vi "Utils.vi"(8 "error in":errorcluster, 10 "Data":variant, 11 "Command":string) -> (0 "error out":errorcluster, 3 "Return Data":variant)   [LabVIEW 2014]
uses:
  <vilib>/Utility/traverseref.llb/TRef TravTarget.ctl
  <vilib>/Utility/traverseref.llb/VI Scripting - Traverse.lvlib
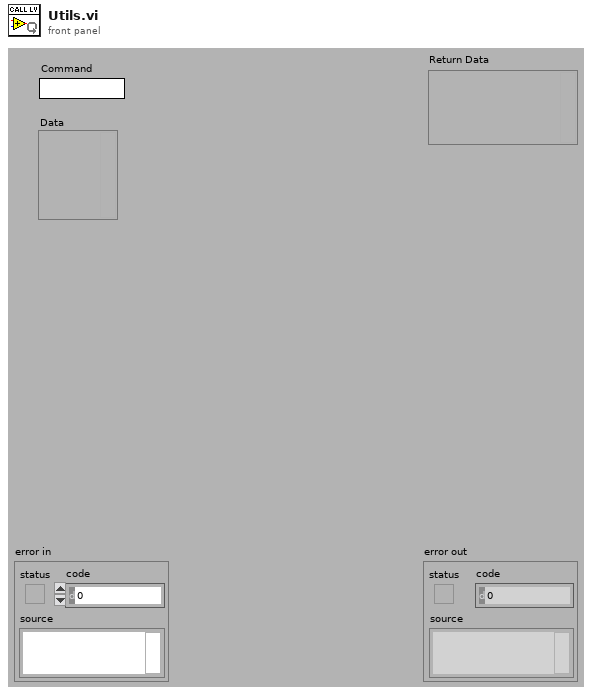
[diagram p1: front panel]
types:
  T1 = typedef "TRef TravTarget.ctl" = enum16{"FP", "BD", "Other"}
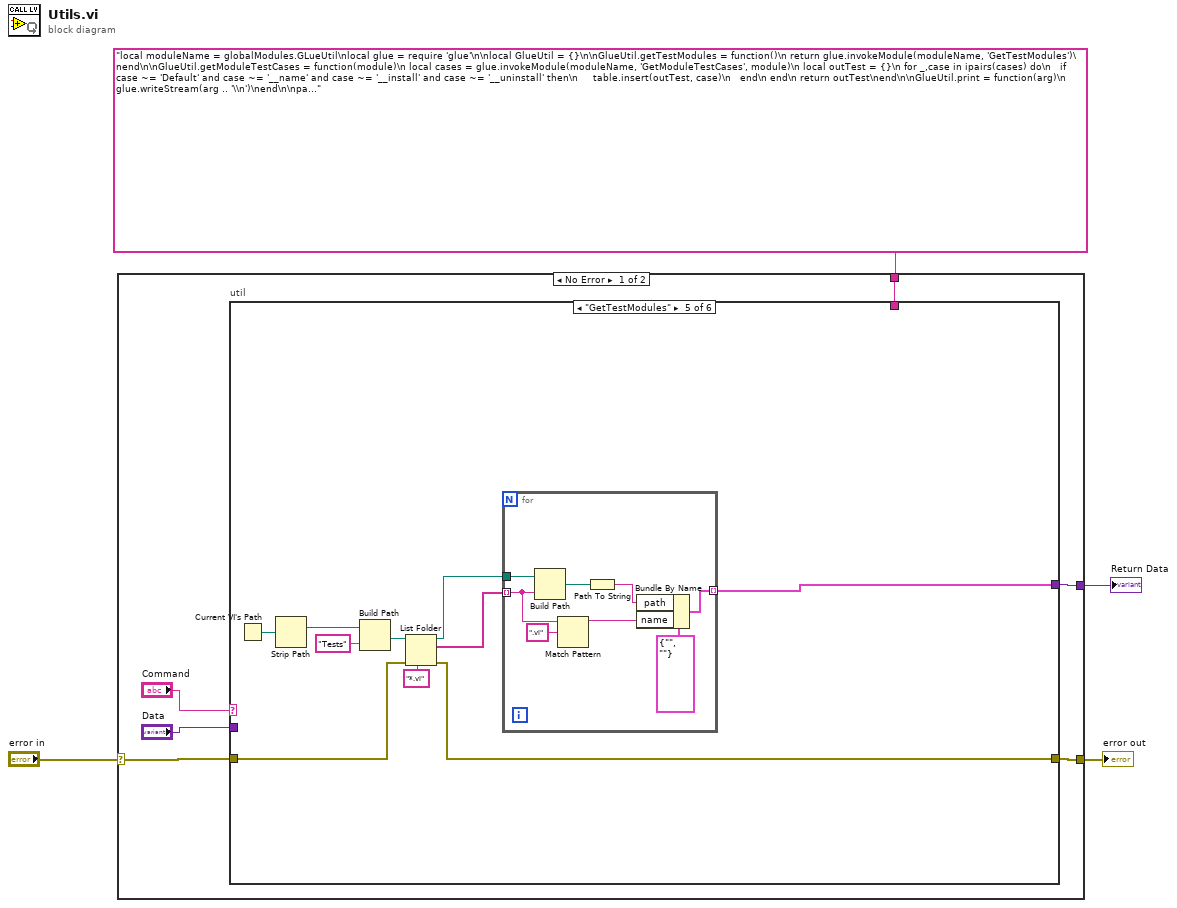
[diagram p0: block diagram]
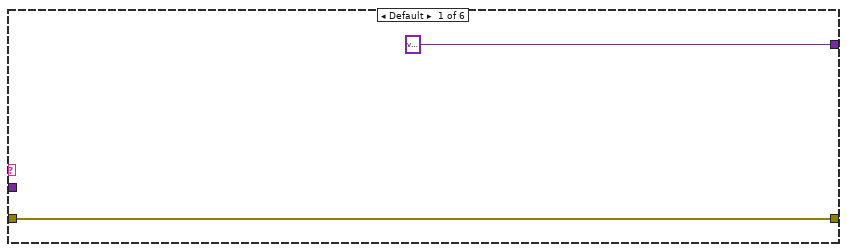
[diagram p2: hidden frame]
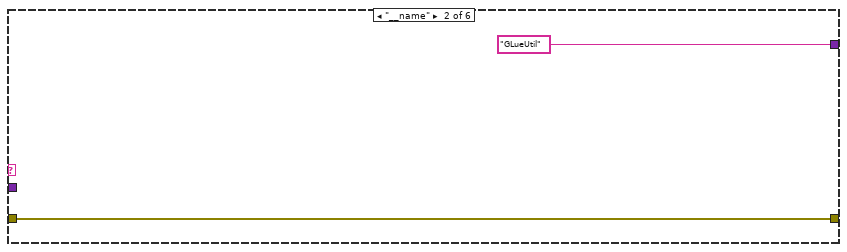
[diagram p3: hidden frame]
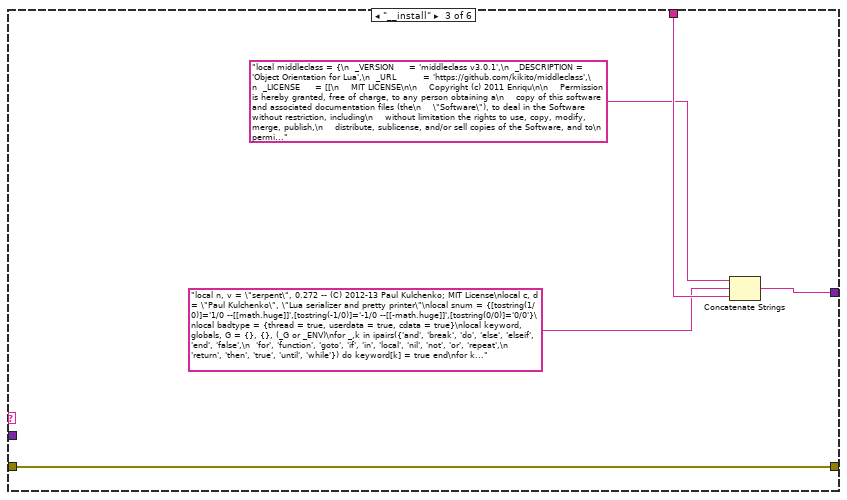
[diagram p4: hidden frame]
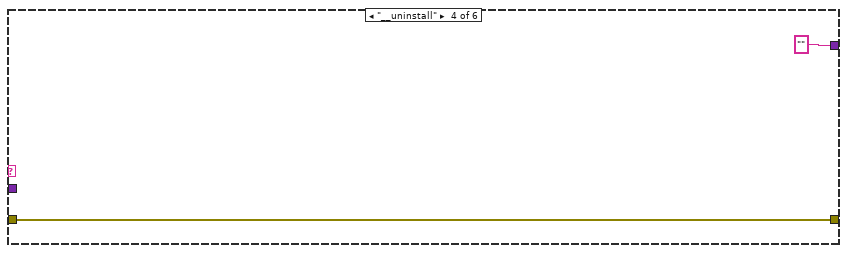
[diagram p5: hidden frame]
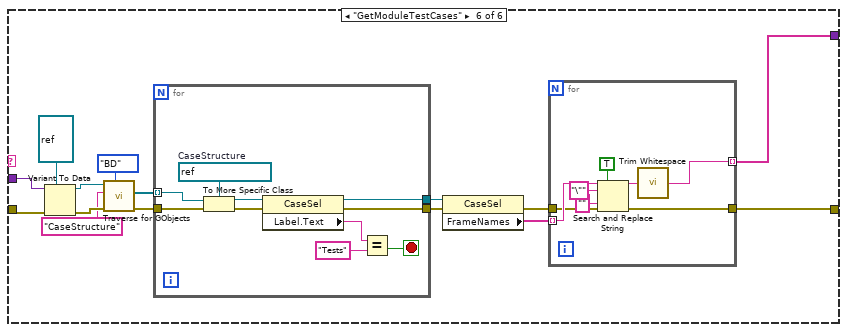
[diagram p6: hidden frame]
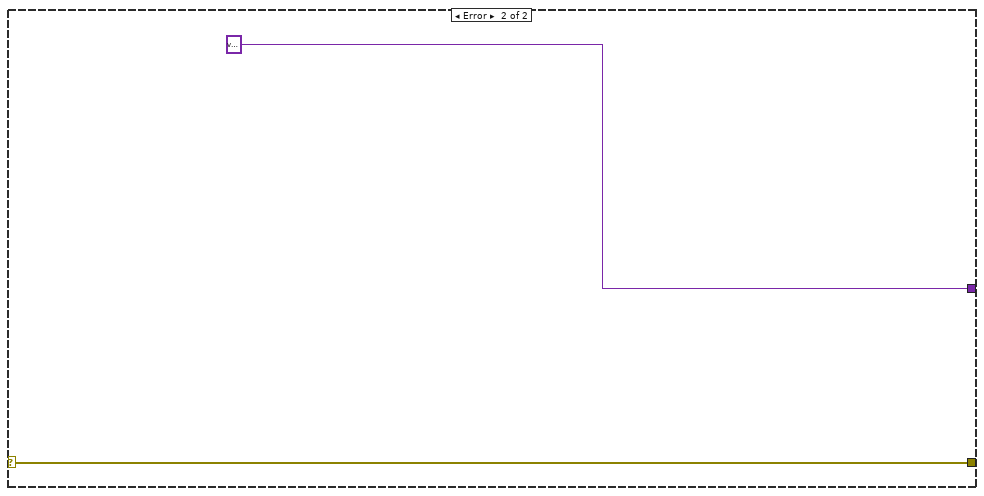
[diagram p7: hidden frame]
diagram:
  n1 = case shown="No Error" "error in" {
    selector: "error in" -> [w10 w74]
    tunnel: [w8 w74] -> w3
    tunnel: [w9 variant ("User Data")] -> w2
    tunnel: "local moduleName = globalModules.GLueUtil\nlocal glue = require 'glue'\n\nlocal GlueUtil = {}\n\nGlueUtil.getTestModules = function()\n return glue.invokeModule(moduleName, 'GetTestModules')\nend\n\nGlueUtil.getModuleTestCases = function(module)\n local cases = glue.invokeModule(moduleName, 'GetModuleTestCases', module)\n local outTest = {}\n for _,case in ipairs(cases) do\n   if case ~= 'Default' and case ~= '__name' and case ~= '__install' and case ~= '__uninstall' then\n     table.insert(outTest, case)\n   end\n end\n return outTest\nend\n\nGlueUtil.print = function(arg)\n  glue.writeStream(arg .. '\\n')\nend\n\npackage.loaded['glueutil'] = GlueUtil" -> [w7 _]
    frame No Error {
      n2 = case "util" shown="\"GetTestModules\"" "Command" {
        tunnel: w10 -> [w12 w13 w19 w20 w27 w54]
        tunnel: "Data" -> [_ _ _ _ _ w44]
        tunnel: [variant ("User Data") "GLueUtil" w17 "" w22 w42] -> w9
        tunnel: [w12 w13 w19 w20 w25 w40] -> w8
        tunnel: w7 -> [_ _ w18 _ _ _]
        frame Default {
        }
        frame "__name" {
        }
        frame "__install" {
          n3 = Concatenate Strings("local middleclass = {\n  _VERSION     = 'middleclass v3.0.1',\n  _DESCRIPTION = 'Object Orientation for Lua',\n  _URL         = 'https://github.com/kikito/middleclass',\n  _LICENSE     = [[\n    MIT LICENSE\n\n    Copyright (c) 2011 Enriqu\n\n    Permission is hereby granted, free of charge, to any person obtaining a\n    copy of this software and associated documentation files (the\n    \"Software\"), to deal in the Software without restriction, including\n    without limitation the rights to use, copy, modify, merge, publish,\n    distribute, sublicense, and/or sell copies of the Software, and to\n    permit persons to whom the Software is furnished to do so, subject to\n    the following conditions:\n\n    The above copyright notice and this permission notice shall be included\n    in all copies or substantial portions of the Software.\n\n    THE SOFTWARE IS PROVIDED \"AS IS\", WITHOUT WARRANTY OF ANY KIND, EXPRESS\n    OR IMPLIED, INCLUDING BUT NOT LIMITED TO THE WARRANTIES OF\n    MERCHANTABILITY, FITNESS FOR A PARTICULAR PURPOSE AND NONINFRINGEMENT.\n    IN NO EVENT SHALL THE AUTHORS OR COPYRIGHT HOLDERS BE LIABLE FOR ANY\n    CLAIM, DAMAGES OR OTHER LIABILITY, WHETHER IN AN ACTION OF CONTRACT,\n    TORT OR OTHERWISE, ARISING FROM, OUT OF OR IN CONNECTION WITH THE\n    SOFTWARE OR THE USE OR OTHER DEALINGS IN THE SOFTWARE.\n  ]]\n}\n\nlocal function _setClassDictionariesMetatables(aClass)\n  local dict = aClass.__instanceDict\n  dict.__index = dict\n\n  local super = aClass.super\n  if super then\n    local superStatic = super.static\n    setmetatable(dict, super.__instanceDict)\n    setmetatable(aClass.static, { __index = function(_,k) return dict[k] or superStatic[k] end })\n  else\n    setmetatable(aClass.static, { __index = function(_,k) return dict[k] end })\n  end\nend\n\nlocal function _setClassMetatable(aClass)\n  setmetatable(aClass, {\n    __tostring = function() return \"class \" .. aClass.name end,\n    __index    = aClass.static,\n    __newindex = aClass.__instanceDict,\n    __call     = function(self, ...) return self:new(...) end\n  })\nend\n\nlocal function _createClass(name, super)\n  local aClass = { name = name, super = super, static = {}, __mixins = {}, __instanceDict={} }\n  aClass.subclasses = setmetatable({}, {__mode = \"k\"})\n\n  _setClassDictionariesMetatables(aClass)\n  _setClassMetatable(aClass)\n\n  return aClass\nend\n\nlocal function _createLookupMetamethod(aClass, name)\n  return function(...)\n    local method = aClass.super[name]\n    assert( type(method)=='function', tostring(aClass) .. \" doesn't implement metamethod '\" .. name .. \"'\" )\n    return method(...)\n  end\nend\n\nlocal function _setClassMetamethods(aClass)\n  for _,m in ipairs(aClass.__metamethods) do\n    aClass[m]= _createLookupMetamethod(aClass, m)\n  end\nend\n\nlocal function _setDefaultInitializeMethod(aClass, super)\n  aClass.initialize = function(instance, ...)\n    return super.initialize(instance, ...)\n  end\nend\n\nlocal function _includeMixin(aClass, mixin)\n  assert(type(mixin)=='table', \"mixin must be a table\")\n  for name,method in pairs(mixin) do\n    if name ~= \"included\" and name ~= \"static\" then aClass[name] = method end\n  end\n  if mixin.static then\n    for name,method in pairs(mixin.static) do\n      aClass.static[name] = method\n    end\n  end\n  if type(mixin.included)==\"function\" then mixin:included(aClass) end\n  aClass.__mixins[mixin] = true\nend\n\nlocal Object = _createClass(\"Object\", nil)\n\nObject.static.__metamethods = { '__add', '__call', '__concat', '__div', '__ipairs', '__le',\n                                '__len', '__lt', '__mod', '__mul', '__pairs', '__pow', '__sub',\n                                '__tostring', '__unm'}\n\nfunction Object.static:allocate()\n  assert(type(self) == 'table', \"Make sure that you are using 'Class:allocate' instead of 'Class.allocate'\")\n  return setmetatable({ class = self }, self.__instanceDict)\nend\n\nfunction Object.static:new(...)\n  local instance = self:allocate()\n  instance:initialize(...)\n  return instance\nend\n\nfunction Object.static:subclass(name)\n  assert(type(self) == 'table', \"Make sure that you are using 'Class:subclass' instead of 'Class.subclass'\")\n  assert(type(name) == \"string\", \"You must provide a name(string) for your class\")\n\n  local subclass = _createClass(name, self)\n  _setClassMetamethods(subclass)\n  _setDefaultInitializeMethod(subclass, self)\n  self.subclasses[subclass] = true\n  self:subclassed(subclass)\n\n  return subclass\nend\n\nfunction Object.static:subclassed(other) end\n\nfunction Object.static:isSubclassOf(other)\n  return type(other)                   == 'table' and\n         type(self)                    == 'table' and\n         type(self.super)              == 'table' and\n         ( self.super == other or\n           type(self.super.isSubclassOf) == 'function' and\n           self.super:isSubclassOf(other)\n         )\nend\n\nfunction Object.static:include( ... )\n  assert(type(self) == 'table', \"Make sure you that you are using 'Class:include' instead of 'Class.include'\")\n  for _,mixin in ipairs({...}) do _includeMixin(self, mixin) end\n  return self\nend\n\nfunction Object.static:includes(mixin)\n  return type(mixin)          == 'table' and\n         type(self)           == 'table' and\n         type(self.__mixins)  == 'table' and\n         ( self.__mixins[mixin] or\n           type(self.super)           == 'table' and\n           type(self.super.includes)  == 'function' and\n           self.super:includes(mixin)\n         )\nend\n\nfunction Object:initialize() end\n\nfunction Object:__tostring() return \"instance of \" .. tostring(self.class) end\n\nfunction Object:isInstanceOf(aClass)\n  return type(self)                == 'table' and\n         type(self.class)          == 'table' and\n         type(aClass)              == 'table' and\n         ( aClass == self.class or\n           type(aClass.isSubclassOf) == 'function' and\n           self.class:isSubclassOf(aClass)\n         )\nend\n\n\n\nfunction middleclass.class(name, super, ...)\n  super = super or Object\n  return super:subclass(name, ...)\nend\n\nmiddleclass.Object = Object\n\nsetmetatable(middleclass, { __call = function(_, ...) return middleclass.class(...) end })\n\npackage.loaded['middleclass'] = middleclass\n", "local n, v = \"serpent\", 0.272 -- (C) 2012-13 Paul Kulchenko; MIT License\nlocal c, d = \"Paul Kulchenko\", \"Lua serializer and pretty printer\"\nlocal snum = {[tostring(1/0)]='1/0 --[[math.huge]]',[tostring(-1/0)]='-1/0 --[[-math.huge]]',[tostring(0/0)]='0/0'}\nlocal badtype = {thread = true, userdata = true, cdata = true}\nlocal keyword, globals, G = {}, {}, (_G or _ENV)\nfor _,k in ipairs({'and', 'break', 'do', 'else', 'elseif', 'end', 'false',\n  'for', 'function', 'goto', 'if', 'in', 'local', 'nil', 'not', 'or', 'repeat',\n  'return', 'then', 'true', 'until', 'while'}) do keyword[k] = true end\nfor k,v in pairs(G) do globals[v] = k end -- build func to name mapping\nfor _,g in ipairs({'coroutine', 'debug', 'io', 'math', 'string', 'table', 'os'}) do\n  for k,v in pairs(G[g] or {}) do globals[v] = g..'.'..k end end\n\nlocal function s(t, opts)\n  local name, indent, fatal, maxnum = opts.name, opts.indent, opts.fatal, opts.maxnum\n  local sparse, custom, huge = opts.sparse, opts.custom, not opts.nohuge\n  local space, maxl = (opts.compact and '' or ' '), (opts.maxlevel or math.huge)\n  local iname, comm = '_'..(name or ''), opts.comment and (tonumber(opts.comment) or math.huge)\n  local seen, sref, syms, symn = {}, {'local '..iname..'={}'}, {}, 0\n  local function gensym(val) return '_'..(tostring(tostring(val)):gsub(\"[^%w]\",\"\"):gsub(\"(%d%w+)\",\n    -- tostring(val) is needed because __tostring may return a non-string value\n    function(s) if not syms[s] then symn = symn+1; syms[s] = symn end return syms[s] end)) end\n  local function safestr(s) return type(s) == \"number\" and (huge and snum[tostring(s)] or s)\n    or type(s) ~= \"string\" and tostring(s) -- escape NEWLINE/010 and EOF/026\n    or (\"%q\"):format(s):gsub(\"\\010\",\"n\"):gsub(\"\\026\",\"\\\\026\") end\n  local function comment(s,l) return comm and (l or 0) < comm and ' --[['..tostring(s)..']]' or '' end\n  local function globerr(s,l) return globals[s] and globals[s]..comment(s,l) or not fatal\n    and safestr(select(2, pcall(tostring, s))) or error(\"Can't serialize \"..tostring(s)) end\n  local function safename(path, name) -- generates foo.bar, foo[3], or foo['b a r']\n    local n = name == nil and '' or name\n    local plain = type(n) == \"string\" and n:match(\"^[%l%u_][%w_]*$\") and not keyword[n]\n    local safe = plain and n or '['..safestr(n)..']'\n    return (path or '')..(plain and path and '.' or '')..safe, safe end\n  local alphanumsort = type(opts.sortkeys) == 'function' and opts.sortkeys or function(k, o, n) -- k=keys, o=originaltable, n=padding\n    local maxn, to = tonumber(n) or 12, {number = 'a', string = 'b'}\n    local function padnum(d) return (\"%0\"..maxn..\"d\"):format(d) end\n    table.sort(k, function(a,b)\n      -- sort numeric keys first: k[key] is not nil for numerical keys\n      return (k[a] ~= nil and 0 or to[type(a)] or 'z')..(tostring(a):gsub(\"%d+\",padnum))\n           < (k[b] ~= nil and 0 or to[type(b)] or 'z')..(tostring(b):gsub(\"%d+\",padnum)) end) end\n  local function val2str(t, name, indent, insref, path, plainindex, level)\n    local ttype, level, mt = type(t), (level or 0), getmetatable(t)\n    local spath, sname = safename(path, name)\n    local tag = plainindex and\n      ((type(name) == \"number\") and '' or name..space..'='..space) or\n      (name ~= nil and sname..space..'='..space or '')\n    if seen[t] then -- already seen this element\n      sref[#sref+1] = spath..space..'='..space..seen[t]\n      return tag..'nil'..comment('ref', level) end\n    if type(mt) == 'table' and (mt.__serialize or mt.__tostring) then -- knows how to serialize itself\n      seen[t] = insref or spath\n      if mt.__serialize then t = mt.__serialize(t) else t = tostring(t) end\n      ttype = type(t) end -- new value falls through to be serialized\n    if ttype == \"table\" then\n      if level >= maxl then return tag..'{}'..comment('max', level) end\n      seen[t] = insref or spath\n      if next(t) == nil then return tag..'{}'..comment(t, level) end -- table empty\n      local maxn, o, out = math.min(#t, maxnum or #t), {}, {}\n      for key = 1, maxn do o[key] = key end\n      if not maxnum or #o < maxnum then\n        local n = #o -- n = n + 1; o[n] is much faster than o[#o+1] on large tables\n        for key in pairs(t) do if o[key] ~= key then n = n + 1; o[n] = key end end end\n      if maxnum and #o > maxnum then o[maxnum+1] = nil end\n      if opts.sortkeys and #o > maxn then alphanumsort(o, t, opts.sortkeys) end\n      local sparse = sparse and #o > maxn -- disable sparsness if only numeric keys (shorter output)\n      for n, key in ipairs(o) do\n        local value, ktype, plainindex = t[key], type(key), n <= maxn and not sparse\n        if opts.valignore and opts.valignore[value] -- skip ignored values; do nothing\n        or opts.keyallow and not opts.keyallow[key]\n        or opts.valtypeignore and opts.valtypeignore[type(value)] -- skipping ignored value types\n        or sparse and value == nil then -- skipping nils; do nothing\n        elseif ktype == 'table' or ktype == 'function' or badtype[ktype] then\n          if not seen[key] and not globals[key] then\n            sref[#sref+1] = 'placeholder'\n            local sname = safename(iname, gensym(key)) -- iname is table for local variables\n            sref[#sref] = val2str(key,sname,indent,sname,iname,true) end\n          sref[#sref+1] = 'placeholder'\n          local path = seen[t]..'['..(seen[key] or globals[key] or gensym(key))..']'\n          sref[#sref] = path..space..'='..space..(seen[value] or val2str(value,nil,indent,path))\n        else\n          out[#out+1] = val2str(value,key,indent,insref,seen[t],plainindex,level+1)\n        end\n      end\n      local prefix = string.rep(indent or '', level)\n      local head = indent and '{\\n'..prefix..indent or '{'\n      local body = table.concat(out, ','..(indent and '\\n'..prefix..indent or space))\n      local tail = indent and \"\\n\"..prefix..'}' or '}'\n      return (custom and custom(tag,head,body,tail) or tag..head..body..tail)..comment(t, level)\n    elseif badtype[ttype] then\n      seen[t] = insref or spath\n      return tag..globerr(t, level)\n    elseif ttype == 'function' then\n      seen[t] = insref or spath\n      local ok, res = pcall(string.dump, t)\n      local func = ok and ((opts.nocode and \"function() --[[..skipped..]] end\" or\n        \"((loadstring or load)(\"..safestr(res)..\",'@serialized'))\")..comment(t, level))\n      return tag..(func or globerr(t, level))\n    else return tag..safestr(t) end -- handle all other types\n  end\n  local sepr = indent and \"\\n\" or \";\"..space\n  local body = val2str(t, name, indent) -- this call also populates sref\n  local tail = #sref>1 and table.concat(sref, sepr)..sepr or ''\n  local warn = opts.comment and #sref>1 and space..\"--[[incomplete output with shared/self-references skipped]]\" or ''\n  return not name and body..warn or \"do local \"..body..sepr..tail..\"return \"..name..sepr..\"end\"\nend\n\nlocal function deserialize(data, opts)\n  local f, res = (loadstring or load)('return '..data)\n  if not f then f, res = (loadstring or load)(data) end\n  if not f then return f, res end\n  if opts and opts.safe == false then return pcall(f) end\n\n  local count, thread = 0, coroutine.running()\n  local h, m, c = debug.gethook(thread)\n  debug.sethook(function (e, l) count = count + 1\n    if count >= 3 then error(\"cannot call functions\") end\n  end, \"c\")\n  local res = {pcall(f)}\n  count = 0 -- set again, otherwise it's tripped on the next sethook\n  debug.sethook(thread, h, m, c)\n  return (table.unpack or unpack)(res)\nend\n\nlocal function merge(a, b) if b then for k,v in pairs(b) do a[k] = v end end; return a; end\nlocal serpent = { _NAME = n, _COPYRIGHT = c, _DESCRIPTION = d, _VERSION = v, serialize = s,\n  load = deserialize,\n  dump = function(a, opts) return s(a, merge({name = '_', compact = true, sparse = true}, opts)) end,\n  line = function(a, opts) return s(a, merge({sortkeys = true, comment = true}, opts)) end,\n  block = function(a, opts) return s(a, merge({indent = '  ', sortkeys = true, comment = true}, opts)) end }\n\npackage.loaded['serpent'] = serpent\n", w18) -> (w17:string)
        }
        frame "__uninstall" {
        }
        frame "GetTestModules" {
          n4 = Current VI's Path() -> (path=w31:path)
          n5 = Strip Path(path=w31) -> (stripped path=w30:path)  [unwired: 1 out]
          n6 = Build Path(base path=w30, name or relative path="Tests") -> (appended path=w28:path)
          n7 = List Folder(path=w28, pattern="*.vi", error in=w27) -> (path out=w26:path, filenames=w23:string[], error out=w25:errorcluster)  [unwired: 1 in, 1 out]
          n8 = for {
            tunnel: w26 -> [w39]
            tunnel: w23 -> [w38] mode=indexing
            tunnel: [w32] -> w22 mode=indexing
            n9 = Build Path(base path=w39, name or relative path=w38) -> (appended path=w36:path)
            n10 = Match Pattern(string=w38, regular expression=".vi") -> (before substring=w34:string)  [unwired: 1 in, 3 out]
            n11 = Path To String(path=w36) -> (string=w33:string)
            n12 = Bundle By Name(cluster=cluster{"name":string, "path":string} {"name"="", "path"=""}, "path"=w33, "name"=w34) -> (w32:cluster{"name":string, "path":string})
          }
        }
        frame "GetModuleTestCases" {
          n13 = Variant To Data(error in=w54, type=refnum<vi> refnum ("This VI"), Variant=w44) -> (data=w52:refnum<vi>, error out=w53:errorcluster)
          n14 = call <vilib>:"Traverse for GObjects.vi"("Traverse Target"=TRef_TravTarget."BD", "error in (no error)"=w53, "Class Name"="CaseStructure", "VI Refnum"=w52) -> ("error out"=w49:errorcluster, "References"=w48:refnum<vi>[])  [unwired: 4 in, 2 out]
          n15 = for {
            tunnel: w49 -> [w71]
            tunnel: w48 -> [w72] mode=indexing
            tunnel: [w67] -> w47
            tunnel: [w63] -> w46
            stop <- w64 stop-if-true
            w70 = refnum<vi> refnum  # CaseStructure
            n16 = To More Specific Class(target class=w70, reference=w72, error in=w71) -> (specific class reference=w69:refnum<vi>, error out=w68:errorcluster)
            n17 = property class="CaseSel"(reference=w69, error in=w68) -> (reference out=w63:refnum<vi>, error out=w67:errorcluster, "Label.Text"=w66:string)
            n18 = Equal?(x=w66, y="Tests") -> (x = y?=w64:bool)
          }
          n19 = property class="CaseSel"(reference=w46, error in=w47) -> (error out=w41:errorcluster, "FrameNames"=w43:string[])  [unwired: 1 out]
          n20 = for {
            tunnel: w43 -> [w62] mode=indexing
            tunnel: [w55] -> w42 mode=indexing
            tunnel: w41 -> [w61]
            tunnel: [w60] -> w40
            n21 = Search and Replace String(replace all?=TRUE ("replace all? (F)"), input string=w62, search string="\"", replace string="" ("replace string (\"\")"), error in=w61) -> (result string=w56:string, error out=w60:errorcluster)  [unwired: 3 in, 2 out]
            n22 = call <vilib>:"Trim Whitespace.vi"("string"=w56) -> ("trimmed string"=w55:string)  [unwired: 1 in]
          }
        }
      }
    }
    frame Error {
    }
  }
  "Return Data" <- w2
  "error out" <- w3
